vi "GetVoltage.vi"(4 "error in":errorcluster, 5 "connection ID":refnum<k5>) -> (0 "Voltage":string, 1 "error out":errorcluster, 2 "connection ID out":refnum<k5>, 3 "Answer":bool)   [LabVIEW 2013]
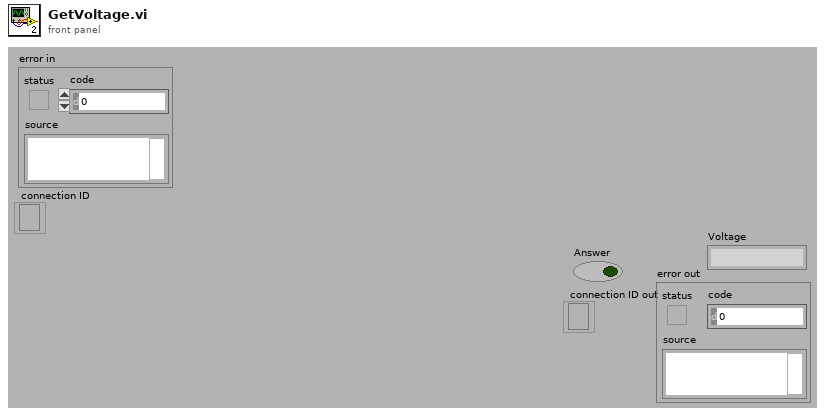
[diagram p1: front panel]
types:
  T1 = enum16{"Standard", "Buffered", "CRLF", "Immediate"}
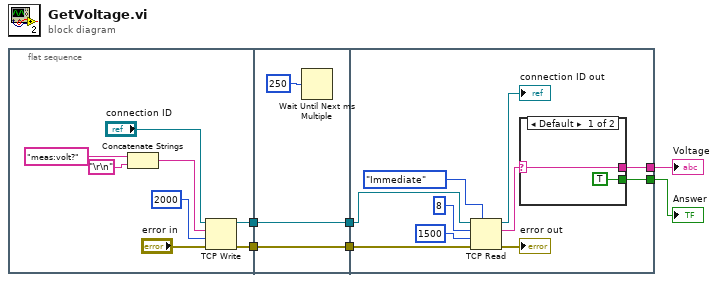
[diagram p0: block diagram]
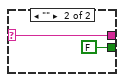
[diagram p2: hidden frame]
diagram:
  n1 = flat-sequence {
    tunnel: [w11] -> w5
    tunnel: [w10] -> w3
    tunnel: [w16] -> w6
    tunnel: w5 -> [w16]
    tunnel: [w15] -> w4
    tunnel: w3 -> [w15]
    tunnel: w6 -> [w21]
    tunnel: w4 -> [w20]
    tunnel: [w19] -> w2
    tunnel: [w18] -> w1
    frame #0 {
      n2 = Concatenate Strings("meas:volt?" ("data in"), "\r\n") -> (w8:string)
      n3 = TCP Write(connection ID="connection ID", data in=w8, error in (no error)="error in", 9:2000 ("timeout ms (25000)")) -> (connection ID out=w11:refnum<k5>, error out=w10:errorcluster)  [unwired: 1 out]
    }
    frame #1 {
      n4 = Wait Until Next ms Multiple(millisecond multiple=u32 250) -> ()  [unwired: 1 out]
    }
    frame #2 {
      n5 = TCP Read(connection ID=w21, bytes to read=8, error in (no error)=w20, 7:T1."Immediate" ("mode (standard)"), 9:1500 ("timeout ms (25000)")) -> (connection ID out=→"connection ID out":refnum<k5>, data out=w25:string, error out=→"error out":errorcluster)
      n6 = case shown="Default" w25 {
        selector: w25 -> [w29 w31]
        tunnel: [w29 w31] -> w19
        tunnel: [TRUE FALSE] -> w18
        frame Default {
        }
        frame "" {
        }
      }
    }
  }
  "Voltage" <- w2
  "Answer" <- w1
